vi "Delay in line(SubVI).vi"(8 "error in (no error)":errorcluster, 10 "milliseconds to wait":u32) -> (0 "error out":errorcluster)   [LabVIEW 2018]
uses:
  <vilib>/LabVIEW Interface for Arduino/Type Defs/Arduino Resource.ctl
  <vilib>/LabVIEW Interface for Arduino/Type Defs/Board Type.ctl
  <vilib>/LabVIEW Interface for Arduino/LabVIEW Interface for Arduino.lvlib
panel:
  in  "Arduino Resource in":T1={"VISA resource"="", "Board Type"=enum."Uno", "Connection Type"=enum."USB / Serial", "Bytes Per Packet (15)"=15}
  out "Arduino Resource Out":T1={"VISA resource"="", "Board Type"=enum."Uno", "Connection Type"=enum."USB / Serial", "Bytes Per Packet (15)"=15}
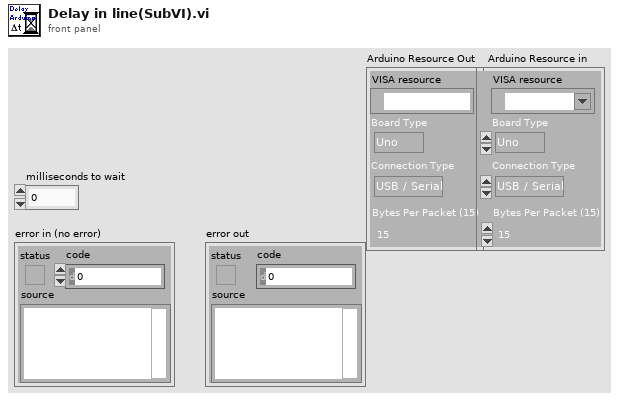
[diagram p1: front panel]
types:
  T1 = typedef "LabVIEW Interface for Arduino.lvlib/Arduino Resource.ctl" = cluster{"VISA resource":refnum<visa-resource-name>, "Board Type":T2, "Connection Type":enum8{"USB / Serial"}, "Bytes Per Packet (15)":u8}
  T2 = typedef "LabVIEW Interface for Arduino.lvlib/Board Type.ctl" = enum16{"Uno", "Dimuelanove w/Atmega 328", "Mega 2560"}
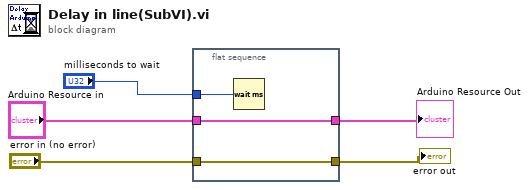
[diagram p0: block diagram]
diagram:
  n1 = flat-sequence {
    tunnel: "milliseconds to wait" -> [w8]
    tunnel: "error in (no error)" -> [w7]
    tunnel: [w7] -> w5
    tunnel: "Arduino Resource in" -> [w6]
    tunnel: [w6] -> w1
    frame #0 {
      n2 = Wait (ms)(milliseconds to wait=w8) -> ()  [unwired: 1 out]
    }
  }
  "error out" <- w5
  "Arduino Resource Out" <- w1
